vi "Set Tree Control Ref.vi"(8 "error in (no error)":errorcluster, 10 "Tree Reference":refnum<vi>, 11 "Process Tree View in":refnum<class "Process Tree View.lvclass">) -> (0 "error out":errorcluster, 3 "Process Tree View out":refnum<class "Process Tree View.lvclass">)   [LabVIEW 2020, in "Process Tree View.lvclass"]
uses:
  Process Tree View.lvclass
  Process Tree View.lvclass/Process Tree View.ctl
  Process Tree View Model/Process Tree View Model.lvclass
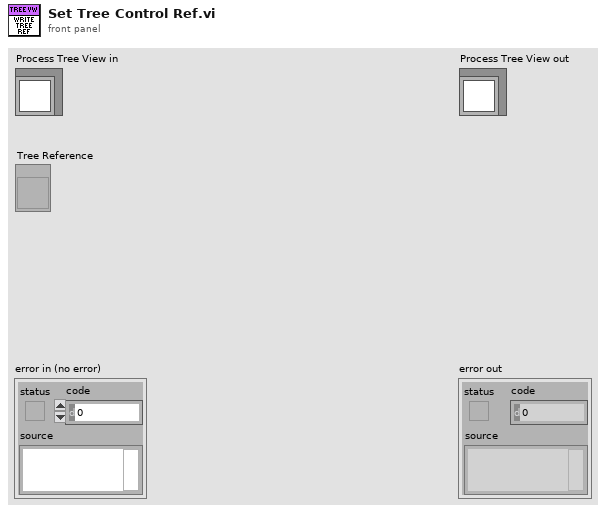
[diagram p1: front panel]
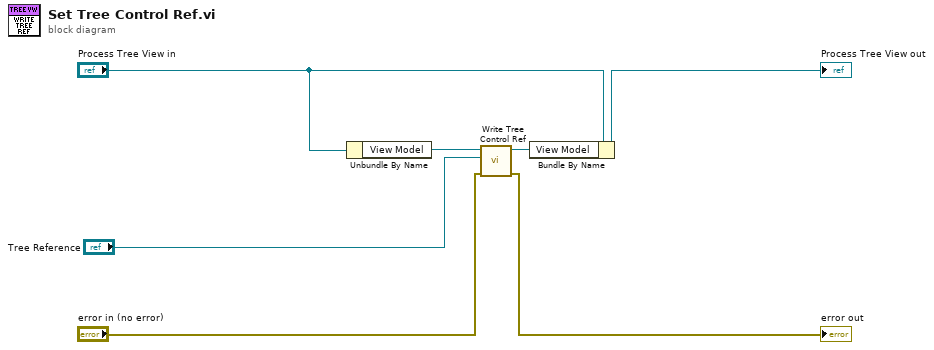
[diagram p0: block diagram]
diagram:
  n1 = Unbundle By Name("Process Tree View in") -> ("View Model"=w6:refnum<class "Process Tree View Model.lvclass">)
  n2 = call "Write Tree Control Ref.vi"("error in (no error)"="error in (no error)", "Tag Tree Reference"="Tree Reference", "Process Tree View Model in"=w6) -> ("error out"=→"error out":errorcluster, "Process Tree View Model out"=w3:refnum<class "Process Tree View Model.lvclass">)  [unwired: 7 in]
  n3 = Bundle By Name(cluster="Process Tree View in", "View Model"=w3) -> (→"Process Tree View out":refnum<class "Process Tree View.lvclass">)
